vi "CRYFFT Filter.vi"(9 "Cutoff Freq":dbl=2.0, 10 "Fs":dbl=2.0, 11 "Signal In":dbl[](array[numeric])) -> (3 "Signal out":dbl[](array[numeric]))   [LabVIEW 2013]
uses:
  <vilib>/Analysis/2dsp.llb/Real FFT.vi
  <vilib>/Analysis/2dsp.llb/Inverse Real FFT.vi
  <vilib>/Analysis/NI_AALPro.lvlib
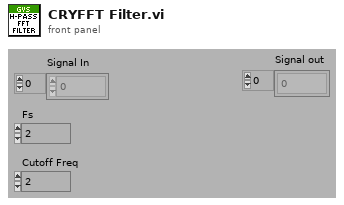
[diagram p1: front panel]
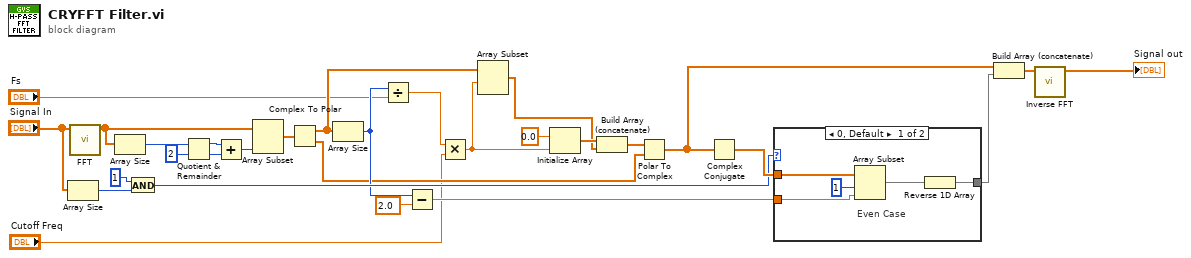
[diagram p0: block diagram]
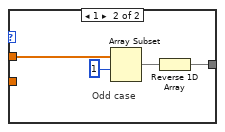
[diagram p2: hidden frame]
diagram:
  n1 = Array Size(array="Signal In") -> (size(s)=w21:i32)
  n2 = call-poly <vilib>:"FFT.vi"("X"="Signal In") -> ("FFT {X}"=w7:cdb[])  [unwired: 9 in, 1 out]
  n3 = Array Size(array=w7) -> (size(s)=w14:i32)
  n4 = And(x=1, y=w21) -> (x .and. y?=w20:i32)
  n5 = Quotient & Remainder(x=w14, y=2) -> (x-y*floor(x/y)=w16:i32, floor(x/y)=w15:i32)
  n6 = Add(x=w16, y=w15) -> (x+y=w13:i32)
  n7 = Array Subset(array=w7, length=w13) -> (w12:cdb[])  [unwired: 1 in]
  n8 = Complex To Polar(r * e^(i*theta)=w12) -> (r=w5:dbl[], theta=w11:dbl[])
  n9 = Array Size(array=w5) -> (size(s)=w19:i32)
  n10 = Divide(x=w19, y="Fs") -> (x/y=w29:dbl)
  n11 = Subtract(x=w19, y=2.0) -> (x-y=w23:dbl)
  n12 = Multiply(x=w29, y="Cutoff Freq") -> (x*y=w18:dbl)
  n13 = Array Subset(array=w5, index=w18) -> (w1:dbl[])  [unwired: 1 in]
  n14 = Initialize Array(0.0 ("element"), w18) -> (w27:dbl[])
  n15 = Build Array (concatenate)(w27, w1) -> (w8:dbl[])
  n16 = Polar To Complex(1:w11, 2:w8) -> (0:w9:cdb[])
  n17 = Complex Conjugate(1:w9) -> (0:w26:cdb[])
  n18 = case shown="0, Default" w20 {
    tunnel: [w34 w35] -> w25
    tunnel: w26 -> [w33 w38]
    tunnel: w23 -> [w30 _]
    frame 0, Default {
      # "Even Case"
      n19 = Array Subset(array=w33, index=1 ("Array Index"), length=w30) -> (w32:cdb[])
      n20 = Reverse 1D Array(array=w32) -> (reversed array=w34:cdb[])
    }
    frame 1 {
      # "Odd case"
      n21 = Array Subset(array=w38, index=1 ("Array Index")) -> (w36:cdb[])  [unwired: 1 in]
      n22 = Reverse 1D Array(array=w36) -> (reversed array=w35:cdb[])
    }
  }
  n23 = Build Array (concatenate)(w9, w25) -> (w10:cdb[])
  n24 = call-poly <vilib>:"Inverse FFT.vi"("FFT {X}"=w10) -> ("X"=→"Signal out":dbl[])  [unwired: 9 in, 1 out]
